vi "PlaMoS_ExecuteSequence.vi"(6 "Total # of seq steps":i32, 8 "error in (no error)":errorcluster, 9 "Curr Iter Params":T9, 10 "PlannedMotionSequence Step":T2={"_Comment"="", "StepParams"={"Ctrl State"=enum."PosCtrl", "CtrlEff Params"={"Time [s]"=0.0, "U_z"=0.0}, "PosCtrl Params"={"Velocity [um/s]"=0.0, "Starting Z-position [um]"=0.0, "Ending Z-position [um]"=0.0, "Bow Reference [um]"=0.0}, "HoldState Params"={"Time [s]"=0.0}}, "Controller Gains"={"Z-direction"={"Kp"=1.0, "Ki"=0.0, "fLPF"=0.0}, "ThX-direction"={"Kp"=0.0, "Ki"=0.0, "fLPF"=0.0}, "ThY-direction"={"Kp"=0.0, "Ki"=0.0, "fLPF"=0.0}, "Bow-direction"={"Kp"=0.0, "Ki"=0.0, "fLPF"=0.0}, "Tor-direction"={"Kp"=0.0, "Ki"=0.0, "fLPF"=0.0}}}, 11 "FPGA VI Reference In":T1) -> (0 "error out":errorcluster, 1 "PlaMoS completed?":bool, 2 "Next State Index":i32, 3 "FPGA VI Reference Out":T1)   [LabVIEW 2020, in "PlannedMotionSequence.lvlib"]
doc: "Generates the setpoints for the Planned Motion Sequence Step, based on the current state index, and current Z-position. Also outputs the next state index for the subsequent iteration.\n\nFPGA I/O are set directly from within the VI."
uses:
  PlannedMotionSequence.lvlib
  TypeDefs/CurrIterParams.ctl
  TypeDefs/PlannedMotionSequence_Step.ctl
  TypeDefs/StepParams.ctl
  TypeDefs/CtrlEff Params.ctl
  TypeDefs/PosCtrl Params.ctl
  TypeDefs/HoldStateParams.ctl
  PC/Controller/TypeDefs/ControllerGains_UI.ctl
  PC/Controller/TypeDefs/ControllerGains_IndAxis.ctl
  FPGA/Components/FPGA TypeDefs/FPGA_Ref_TypeDef.ctl
  Timing/Timing Action Engine/TimingCmd Enum.ctl
  Timing/Timing Action Engine/Timing Action Engine.lvlib
  RT Target/Controller/Components/FPGA control IO/FPGAcontrolIO.lvlib
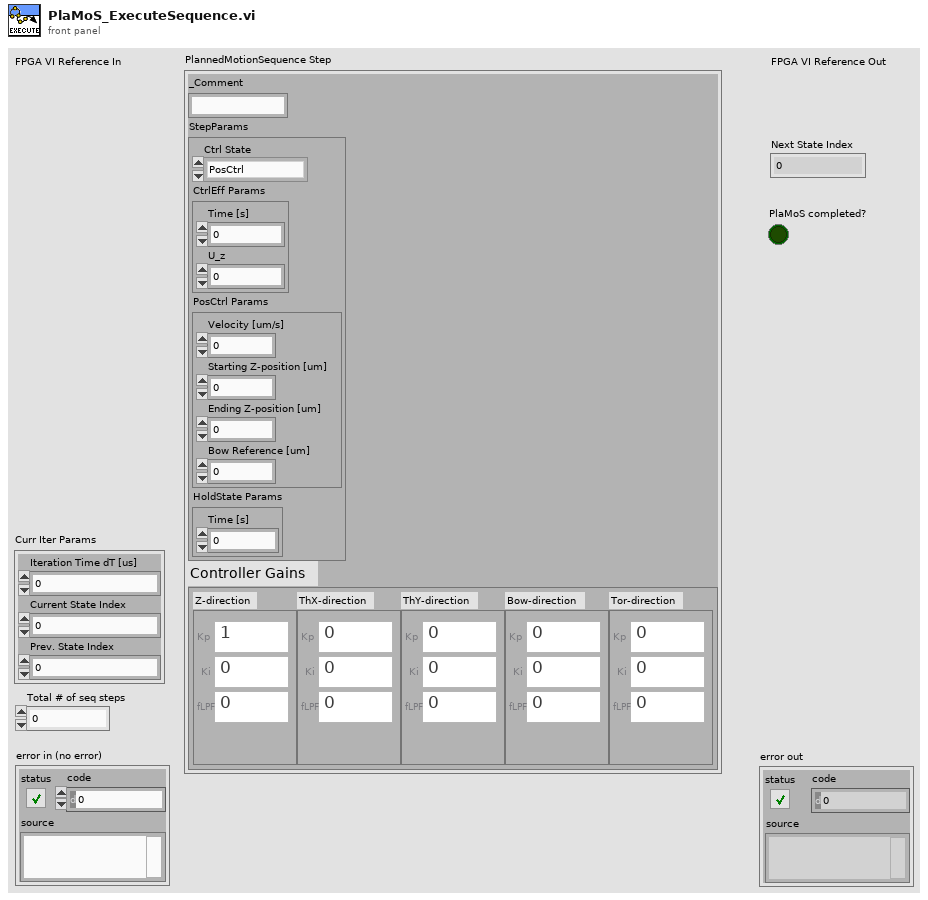
[diagram p1: front panel]
types:
  T1 = typedef "FPGA_Ref_TypeDef.ctl" = refnum<k20>
  T2 = typedef "PlannedMotionSequence.lvlib/PlannedMotionSequence_Step.ctl" = cluster{"_Comment":string, "StepParams":T3, "Controller Gains":T7}
  T3 = typedef "PlannedMotionSequence.lvlib/StepParams.ctl" = cluster{"Ctrl State":enum16{"PosCtrl", "CtrlEff", "HoldState"}, "CtrlEff Params":T4, "PosCtrl Params":T5, "HoldState Params":T6}
  T4 = typedef "PlannedMotionSequence.lvlib/CtrlEff Params.ctl" = cluster{"Time [s]":dbl, "U_z":dbl}
  T5 = typedef "PlannedMotionSequence.lvlib/PosCtrl Params.ctl" = cluster{"Velocity [um/s]":dbl, "Starting Z-position [um]":dbl, "Ending Z-position [um]":dbl, "Bow Reference [um]":dbl}
  T6 = typedef "PlannedMotionSequence.lvlib/HoldStateParams.ctl" = cluster{"Time [s]":dbl}
  T7 = typedef "ControllerGains_UI.ctl" = cluster{"Z-direction":T8, "ThX-direction":T8, "ThY-direction":T8, "Bow-direction":T8, "Tor-direction":T8}
  T8 = typedef "ControllerGains_IndAxis.ctl" = cluster{"Kp":dbl, "Ki":dbl, "fLPF":dbl}
  T9 = typedef "PlannedMotionSequence.lvlib/CurrIterParams.ctl" = cluster{"Iteration Time dT [us]":dbl, "Current State Index":i32, "Prev. State Index":i32}
  T10 = typedef "Timing.lvlib/Timing Action Engine.lvlib/TimingCmd Enum.ctl" = enum16{"Reset", "Pause", "Read Time"}
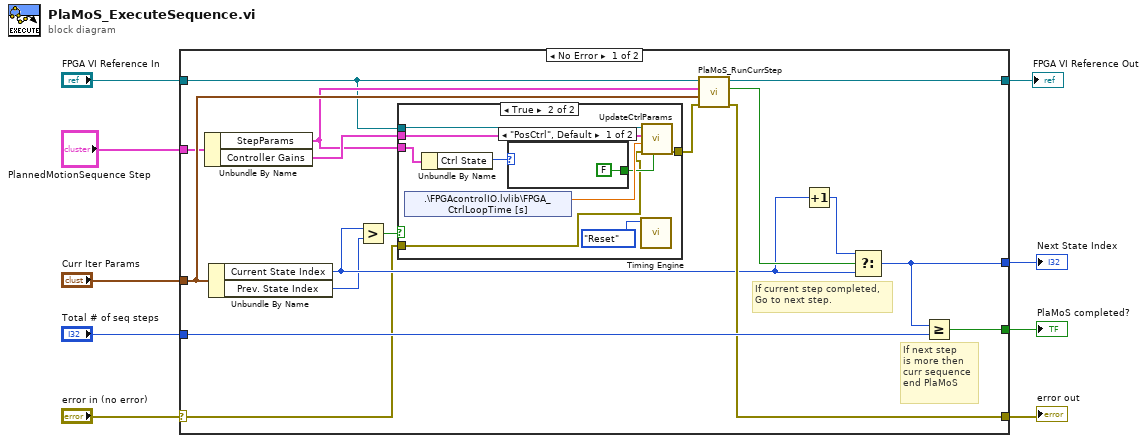
[diagram p0: block diagram]
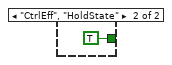
[diagram p3: hidden frame]
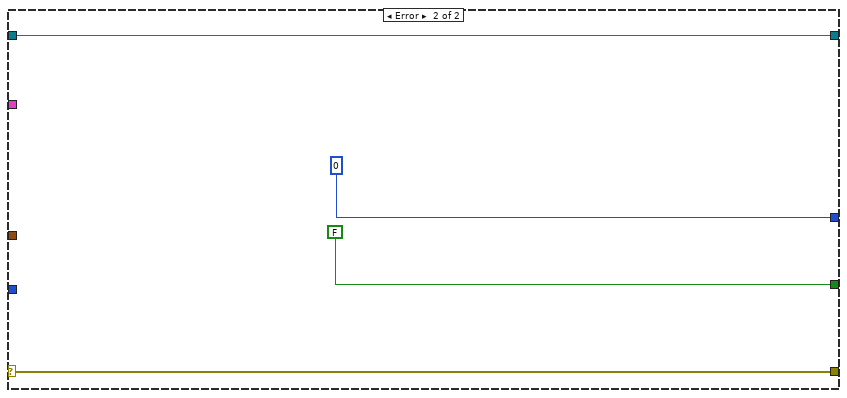
[diagram p4: hidden frame]
diagram:
  n1 = case shown="No Error" "error in (no error)" {
    selector: "error in (no error)" -> [w13 w42]
    tunnel: [w21 w42] -> w8
    tunnel: "FPGA VI Reference In" -> [w11 w41]
    tunnel: [w10 w41] -> w1
    tunnel: "Curr Iter Params" -> [w20 _]
    tunnel: [w24 0 ("Current State Index")] -> w6
    tunnel: [w23 FALSE] -> w5
    tunnel: "Total # of seq steps" -> [w22 _]
    tunnel: "PlannedMotionSequence Step" -> [w19 _]
    frame No Error {
      # "If next step\nis more then\ncurr sequence\nend PlaMoS"
      # "If current step completed,\nGo to next step."
      n2 = Unbundle By Name(w19) -> ("StepParams"=w14:T3, "Controller Gains"=w15:T7)
      n3 = Unbundle By Name(w20) -> ("Current State Index"=w17:i32, "Prev. State Index"=w16:i32)
      n4 = Greater?(x=w17, y=w16) -> (0:w18:bool)
      n5 = case shown="True" w18 {
        tunnel: w11 -> [_ w34]
        tunnel: w15 -> [_ w33]
        tunnel: w14 -> [_ w32]
        tunnel: w13 -> [w27 w29]
        tunnel: [w27 w28] -> w12
        frame False {
        }
        frame True {
          n6 = shared-variable ".\\FPGAcontrolIO.lvlib\\FPGA_CtrlLoopTime [s]"() -> (w35:dbl)  [unwired: 1 in, 1 out]
          n7 = Unbundle By Name(w32) -> ("Ctrl State"=w31:enum16{"PosCtrl", "CtrlEff", "HoldState"})
          n8 = case shown="\"PosCtrl\", Default" w31 {
            tunnel: [FALSE TRUE] -> w30
            frame "PosCtrl", Default {
            }
            frame "CtrlEff", "HoldState" {
            }
          }
          n9 = call "Timing Engine.vi"("Timing Cmd In"=TimingCmd_Enum."Reset") -> ()  [unwired: 8 in, 3 out]
          n10 = call "UpdateCtrlParams.vi"("Ignore Update? (F)"=w30, "error in (no error)"=w29, "Ts [s]"=w35, "Controller Gains"=w33, "FPGA VI Reference In"=w34) -> ("error out"=w28:errorcluster)  [unwired: 5 in, 1 out]
        }
      }
      n11 = call "PlaMoS_RunCurrStep.vi"("error in (no error)"=w12, "Curr Iter Params"=w20, "StepParams"=w14, "FPGA VI Reference In"=w11) -> ("error out"=w21:errorcluster, "Step Completed?"=w26:bool, "FPGA VI Reference Out"=w10:T1)  [unwired: 5 in]
      n12 = Increment(x=w17) -> (x+1=w25:i32)
      n13 = Select(t=w25, s=w26, f=w17) -> (s? t:f=w24:i32)
      n14 = Greater Or Equal?(x=w24, y=w22) -> (x >= y?=w23:bool)
    }
    frame Error {
    }
  }
  "error out" <- w8
  "Next State Index" <- w6
  "PlaMoS completed?" <- w5
  "FPGA VI Reference Out" <- w1
